vi "Calculate data.vi"(0 "D IO":u16, 1 "Criteria":T1, 5 "A IO":u16, 7 "A IO 1":u16, 9 "A IO 2":u16, 11 "Limit in main":bool, 12 "Limit analog 1":dbl, 13 "Limit analog 2":dbl, 14 "Time":dbl) -> (8 "Data":T2)   [LabVIEW 2011, in "Criteria control.xctl"]
uses:
  Criteria control.xctl
  Data 3.ctl
  Single criteria cluster.ctl
  Criteria types.ctl
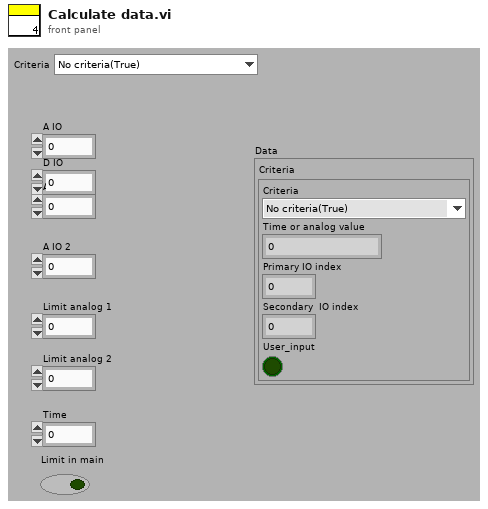
[diagram p1: front panel]
types:
  T1 = typedef "Criteria types.ctl" = enum16{"No criteria(True)", "Time(s)", "Analog IO over", "Analog IO over or equal", "Analog IO under", "Analog IO under or equal", "Analog IO 1 minus Analog IO 2 over", "Digital IO True", "Digital IO False", "Operator approval"}
  T2 = typedef "Criteria control.xctl/Data 3.ctl" = cluster{"Criteria":T3}
  T3 = typedef "Single criteria cluster.ctl" = cluster{"Criteria":T1, "Time or analog value":dbl, "Primary IO index":i32, "Secondary  IO index":i32, "User_input":bool}
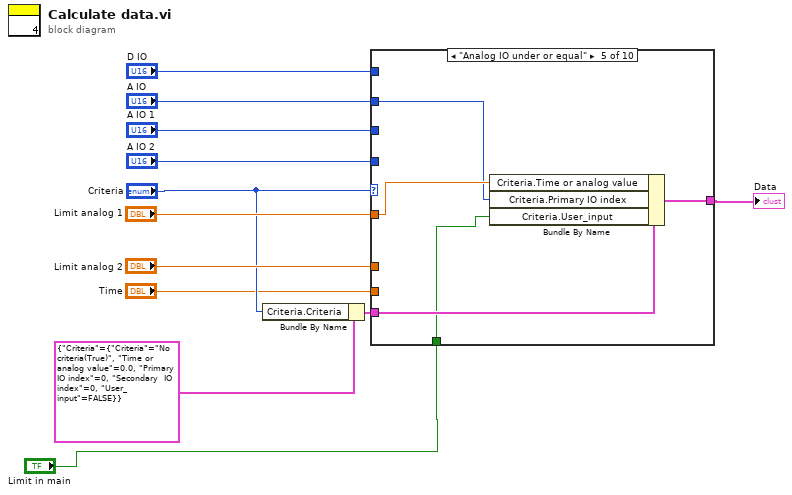
[diagram p0: block diagram]
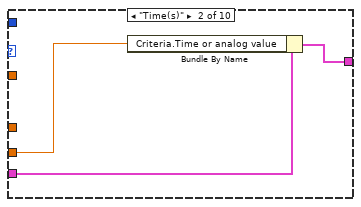
[diagram p3: hidden frame]
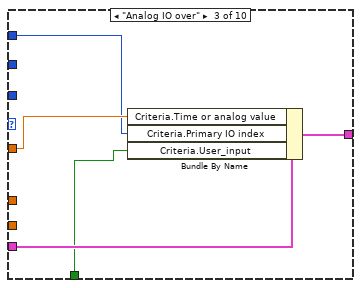
[diagram p4: hidden frame]
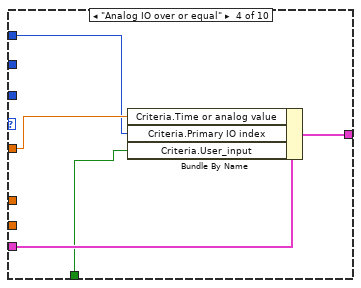
[diagram p5: hidden frame]
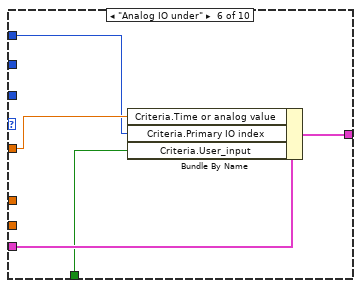
[diagram p6: hidden frame]
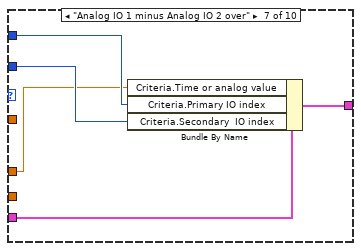
[diagram p7: hidden frame]
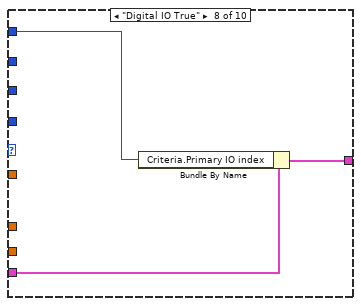
[diagram p8: hidden frame]
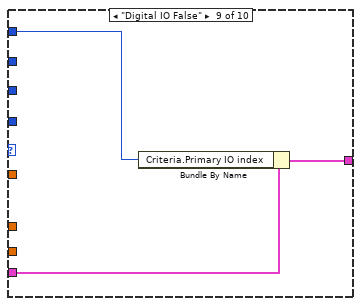
[diagram p9: hidden frame]
diagram:
  n1 = Bundle By Name(cluster=T2 {"Criteria"={"Criteria"=enum."No criteria(True)", "Time or analog value"=0.0, "Primary IO index"=0, "Secondary  IO index"=0, "User_input"=FALSE}} ("Data In"), "Criteria.Criteria"="Criteria") -> (w4:T2)
  n2 = case shown="\"Analog IO under or equal\"" "Criteria" {
    tunnel: "Limit analog 1" -> [_ _ w19 w24 w29 w34 _ _ _ _]
    tunnel: "A IO 1" -> [_ _ _ _ _ _ w38 _ _ _]
    tunnel: "A IO 2" -> [_ _ _ _ _ _ w39 _ _ _]
    tunnel: [w13 w15 w20 w25 w30 w35 w40 w43 w46 w48] -> w12
    tunnel: "Limit analog 2" -> [_ _ _ _ _ _ w37 _ _ _]
    tunnel: "D IO" -> [_ _ _ _ _ _ _ w42 w45 _]
    tunnel: "A IO" -> [_ _ w18 w23 w28 w33 _ _ _ _]
    tunnel: w4 -> [w13 w16 w21 w26 w31 w36 w41 w44 w47 w48]
    tunnel: "Time" -> [_ w14 _ _ _ _ _ _ _ _]
    tunnel: "Limit in main" -> [_ _ w17 w22 w27 w32 _ _ _ _]
    frame "No criteria(True)", Default {
    }
    frame "Time(s)" {
      n3 = Bundle By Name(cluster=w16, "Criteria.Time or analog value"=w14) -> (w15:T2)
    }
    frame "Analog IO over" {
      n4 = Bundle By Name(cluster=w21, "Criteria.Time or analog value"=w19, "Criteria.Primary IO index"=w18, "Criteria.User_input"=w17) -> (w20:T2)
    }
    frame "Analog IO over or equal" {
      n5 = Bundle By Name(cluster=w26, "Criteria.Time or analog value"=w24, "Criteria.Primary IO index"=w23, "Criteria.User_input"=w22) -> (w25:T2)
    }
    frame "Analog IO under or equal" {
      n6 = Bundle By Name(cluster=w31, "Criteria.Time or analog value"=w29, "Criteria.Primary IO index"=w28, "Criteria.User_input"=w27) -> (w30:T2)
    }
    frame "Analog IO under" {
      n7 = Bundle By Name(cluster=w36, "Criteria.Time or analog value"=w34, "Criteria.Primary IO index"=w33, "Criteria.User_input"=w32) -> (w35:T2)
    }
    frame "Analog IO 1 minus Analog IO 2 over" {
      n8 = Bundle By Name(cluster=w41, "Criteria.Time or analog value"=w37, "Criteria.Primary IO index"=w38, "Criteria.Secondary  IO index"=w39) -> (w40:T2)
    }
    frame "Digital IO True" {
      n9 = Bundle By Name(cluster=w44, "Criteria.Primary IO index"=w42) -> (w43:T2)
    }
    frame "Digital IO False" {
      n10 = Bundle By Name(cluster=w47, "Criteria.Primary IO index"=w45) -> (w46:T2)
    }
    frame "Operator approval" {
    }
  }
  "Data" <- w12
